vi "CheckBacklogQueue.vi"(7 "Qbus":refnum<class "Qbus.lvclass">, 8 "error in (no error)":errorcluster, 11 "BacklogQ":refnum<queue>) -> (0 "error out":errorcluster, 2 "ready":bool, 3 "data":variant)   [LabVIEW 2017, in "FileManager.lvlib"]
uses:
  <vilib>/addons/InsightCM/Devices/Shared/Common/FileManager/FileManager.lvlib
  <vilib>/addons/Qbus/Qbus.lvclass
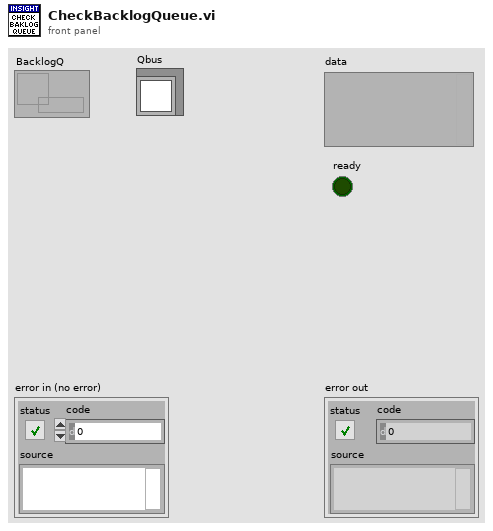
[diagram p1: front panel]
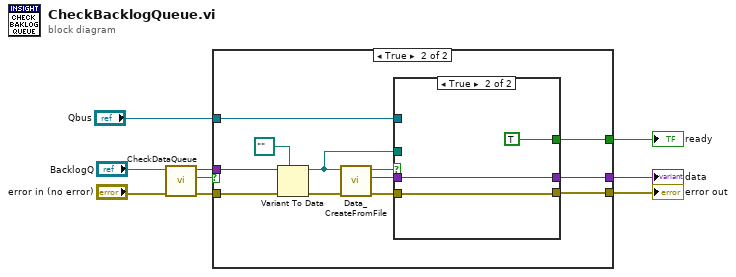
[diagram p0: block diagram]
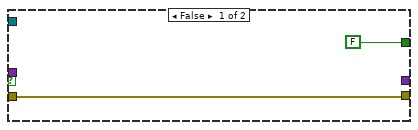
[diagram p2: hidden frame]
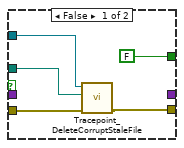
[diagram p3: hidden frame]
diagram:
  n1 = call <vilib>:"CheckDataQueue.vi"("error in (no error)"="error in (no error)", "data Q"="BacklogQ") -> ("error out"=w7:errorcluster, "ready"=w4:bool, "data"=w6:variant)  [unwired: 7 in]
  n2 = case shown="True" w4 {
    tunnel: w7 -> [w10 w23]
    tunnel: w6 -> [_ w22]
    tunnel: [_ w17] -> w5
    tunnel: "Qbus" -> [_ w14]
    tunnel: [w10 w13] -> w2
    tunnel: [FALSE w12] -> w1
    frame False {
    }
    frame True {
      n3 = Variant To Data(error in=w23, type=path "", Variant=w22) -> (data=w15:path, error out=w21:errorcluster)
      n4 = call <vilib>:"Data_CreateFromFile.vi"("error in (no error)"=w21, "Path"=w15) -> ("error out"=w19:errorcluster, "data"=w16:variant, "success"=w18:bool)  [unwired: 7 in]
      n5 = case shown="True" w18 {
        tunnel: w19 -> [w28 w30]
        tunnel: [_ w31] -> w17
        tunnel: w16 -> [_ w31]
        tunnel: w15 -> [w27 _]
        tunnel: w14 -> [w26 _]
        tunnel: [w25 w30] -> w13
        tunnel: [FALSE TRUE] -> w12
        frame False {
          n6 = call <vilib>:"Tracepoint_DeleteCorruptStaleFile.vi"("error in (no error)"=w28, "file"=w27, "Qbus in"=w26) -> ("error out"=w25:errorcluster)  [unwired: 8 in]
        }
        frame True {
        }
      }
    }
  }
  "error out" <- w2
  "data" <- w5
  "ready" <- w1
